vi "Parse Stored String.vi"(1 "stored string":string) -> (0 "parsed string":string)   [LabVIEW 2009]
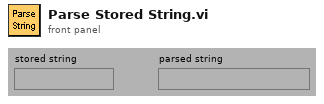
[diagram p1: front panel]
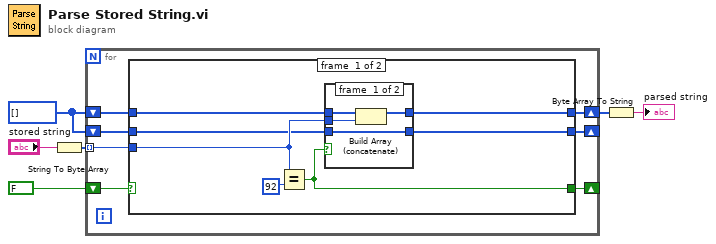
[diagram p0: block diagram]
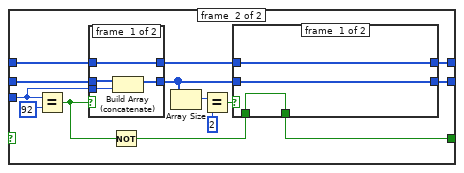
[diagram p3: hidden frame]
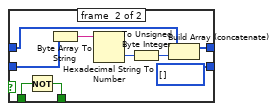
[diagram p4: hidden frame]
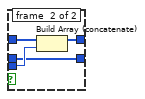
[diagram p5: hidden frame]
diagram:
  w1 = u8[] []
  n1 = String To Byte Array(string="stored string") -> (unsigned byte array=w3:u8[])
  n2 = for {
    tunnel: w3 -> [w9] mode=indexing
    shift-right: [w12] -> w4
    shift-left: w1 -> [w13]
    shift-right: [w10] -> _
    shift-left: FALSE -> [w11]
    shift-right: [w7] -> _
    shift-left: w1 -> [w8]
    n3 = case shown="True" w11 {
      tunnel: w13 -> [w18 w40]
      tunnel: [w17 w30] -> w12
      tunnel: [w19 w28] -> w10
      tunnel: w9 -> [w16 w27]
      tunnel: w8 -> [w15 w37]
      tunnel: [w14 w32] -> w7
      frame #0 {
        n4 = Equal?(x=w16, y=u8 92) -> (x = y?=w19:bool)
        n5 = case shown="False" w19 {
          tunnel: [w23 w26] -> w17
          tunnel: w18 -> [w24 w26]
          tunnel: w16 -> [w22 _]
          tunnel: [w21 w25] -> w14
          tunnel: w15 -> [w21 w25]
          frame #0 {
            n6 = Build Array (concatenate)(w24, w22) -> (w23:u8[])
          }
          frame #1 {
          }
        }
      }
      frame #1 {
        n7 = Equal?(x=w27, y=u8 92) -> (x = y?=w38:bool)
        n8 = case shown="False" w38 {
          tunnel: w40 -> [w56 w60]
          tunnel: [w56 w59] -> w31
          tunnel: w27 -> [w54 w58]
          tunnel: [w53 w57] -> w33
          tunnel: w37 -> [w55 w57]
          frame #0 {
            n9 = Build Array (concatenate)(w55, w54) -> (w53:u8[])
          }
          frame #1 {
            n10 = Build Array (concatenate)(w60, w58) -> (w59:u8[])
          }
        }
        n11 = Not(x=w38) -> (.not. x?=w29:bool)
        n12 = Array Size(array=w33) -> (size(s)=w36:i32)
        n13 = Equal?(x=w36, y=2) -> (x = y?=w34:bool)
        n14 = case shown="True" w34 {
          tunnel: [w43 u8[] []] -> w32
          tunnel: w33 -> [w43 w51]
          tunnel: [w42 w45] -> w30
          tunnel: w31 -> [w42 w47]
          tunnel: w29 -> [w41 w50]
          tunnel: [w41 w49] -> w28
          frame #0 {
          }
          frame #1 {
            n15 = Not(x=w50) -> (.not. x?=w49:bool)
            n16 = Byte Array To String(unsigned byte array=w51) -> (string=w48:string)
            n17 = Hexadecimal String To Number(string=w48) -> (number=w46:u32)  [unwired: 2 in, 1 out]
            n18 = To Unsigned Byte Integer(number=w46) -> (unsigned 8bit integer=w44:u8)
            n19 = Build Array (concatenate)(w47, w44) -> (w45:u8[])
          }
        }
      }
    }
  }
  n20 = Byte Array To String(unsigned byte array=w4) -> (string=→"parsed string":string)
